vi "烧录座显示界面.vi"(8 "错误输入（无错误）":errorcluster, 10 "界面切换队列":refnum<queue>, 11 "VISA资源名称输入":refnum<visa-resource-name>) -> (0 "错误输出":errorcluster, 3 "VISA资源名称输出":refnum<visa-resource-name>)   [LabVIEW 2018]
panel:
  out "毫秒计时值":u32
  in  "枚举":T1(ring)
  in  "选项卡控件":enum32{"选项卡 1", "选项卡 2"}(tab)
  out "烧录座设定界面":bool
  out "读DDT32250+写R890":dbl
  out "读DDT32252+写R891":dbl
  out "读DDT32254+写R892":dbl
  out "读DDT32256+写R893":dbl
  out "读DDT32258+写R894":dbl
  out "读DDT32260+写R895":dbl
  out "读DDT32262+写R896":dbl
  out "读DDT32264+写R897":dbl
  out "读DDT32266+写R898":dbl
  out "读DDT32268+写R899":dbl
  out "读DDT32270+写R89A":dbl
  out "读DDT32272+写R89B":dbl
  out "读DDT32274+写R89C":dbl
  out "读DDT32276+写R89D":dbl
  out "读DDT32278+写R89E":dbl
  out "读DDT32280+写R89F":dbl
  out "DDT90356":dbl
  out "DDT90348":dbl
  out "自动界面":bool
  out "手动界面":bool
  out "参数界面":bool
  out "IO界面":bool
  out "产品界面":bool
  out "字符串":string
  out "DDT90352":dbl
  out "DDT90360":dbl
  out "通讯周期":dbl
  out "DT1184":T2(ring)
  out "读DDT32200+写R880":dbl
  out "读DDT32202+写R881":dbl
  out "读DDT32204+写R882":dbl
  out "读DDT32206+写R883":dbl
  out "读DDT32208+写R884":dbl
  out "读DDT32210+写R885":dbl
  out "读DDT32212+写R886":dbl
  out "读DDT32214+写R887":dbl
  out "读DDT32216+写R888":dbl
  out "读DDT32218+写R889":dbl
  out "读DDT32220+写R88A":dbl
  out "读DDT32222+写R88B":dbl
  out "读DDT32224+写R88C":dbl
  out "读DDT32226+写R88D":dbl
  out "读DDT32228+写R88E":dbl
  out "读DDT32230+写R88F":dbl
  # "X"
  # "Z1"
  # "Z2"
  # "Y"
  # "1"
  # "2"
  # "3"
  # "4"
  # "5"
  # "6"
  # "7"
  # "8"
  # "9"
  # "10"
  # "12"
  # "14"
  # "15"
  # "16"
  # "11"
  # "13"
  # "烧录座当前OK数量"
  # "鼠标点击数值框清零"
  # "1"
  # "2"
  # "3"
  # "4"
  # "5"
  # "6"
  # "7"
  # "8"
  # "9"
  # "10"
  # "12"
  # "14"
  # "15"
  # "16"
  # "11"
  # "13"
  # "烧录座当前NG数量"
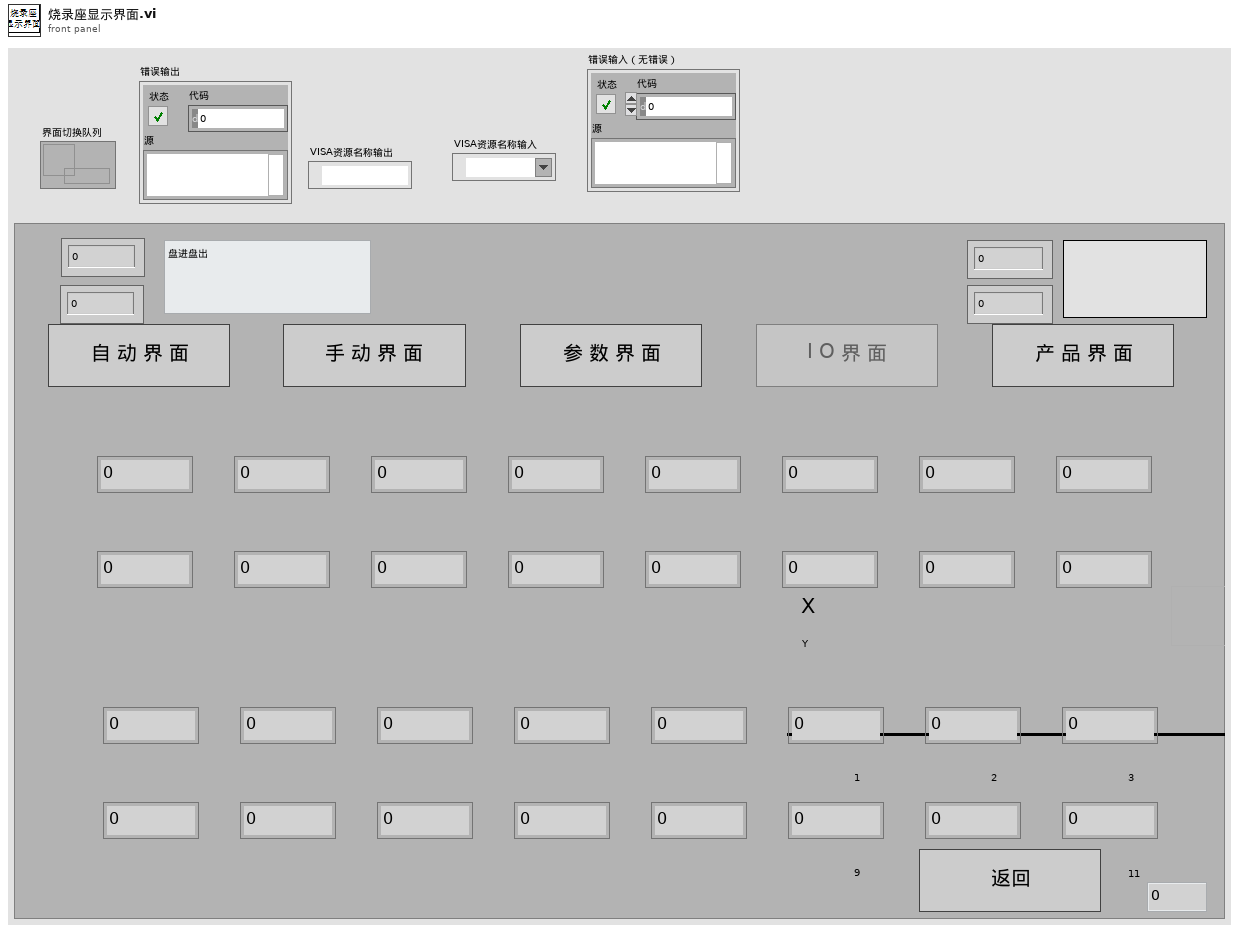
[diagram p1: front panel]
types:
  T1 = enum16{"读初始化", "读DDT32230", "读DDT32220+5", "读DDT32210+5", "读DDT32200+5", "读DDT32280", "读DDT32270+5", "读DDT32260+5", "读DDT32250+5", "读DDT90356", "读DT1184", "读DDT90348", ""}
  T2 = enum16{"盘进盘出", "卷进卷出", "盘进卷出", "管进盘出", "管进卷出", "卷进盘出", ""}
  T3 = enum8{"Enabled", "Disabled", "Disabled and Grayed Out"}
  T4 = typedef "数据簇.ctl" = cluster{"字符串":string, "数值":i32, "布尔":bool}
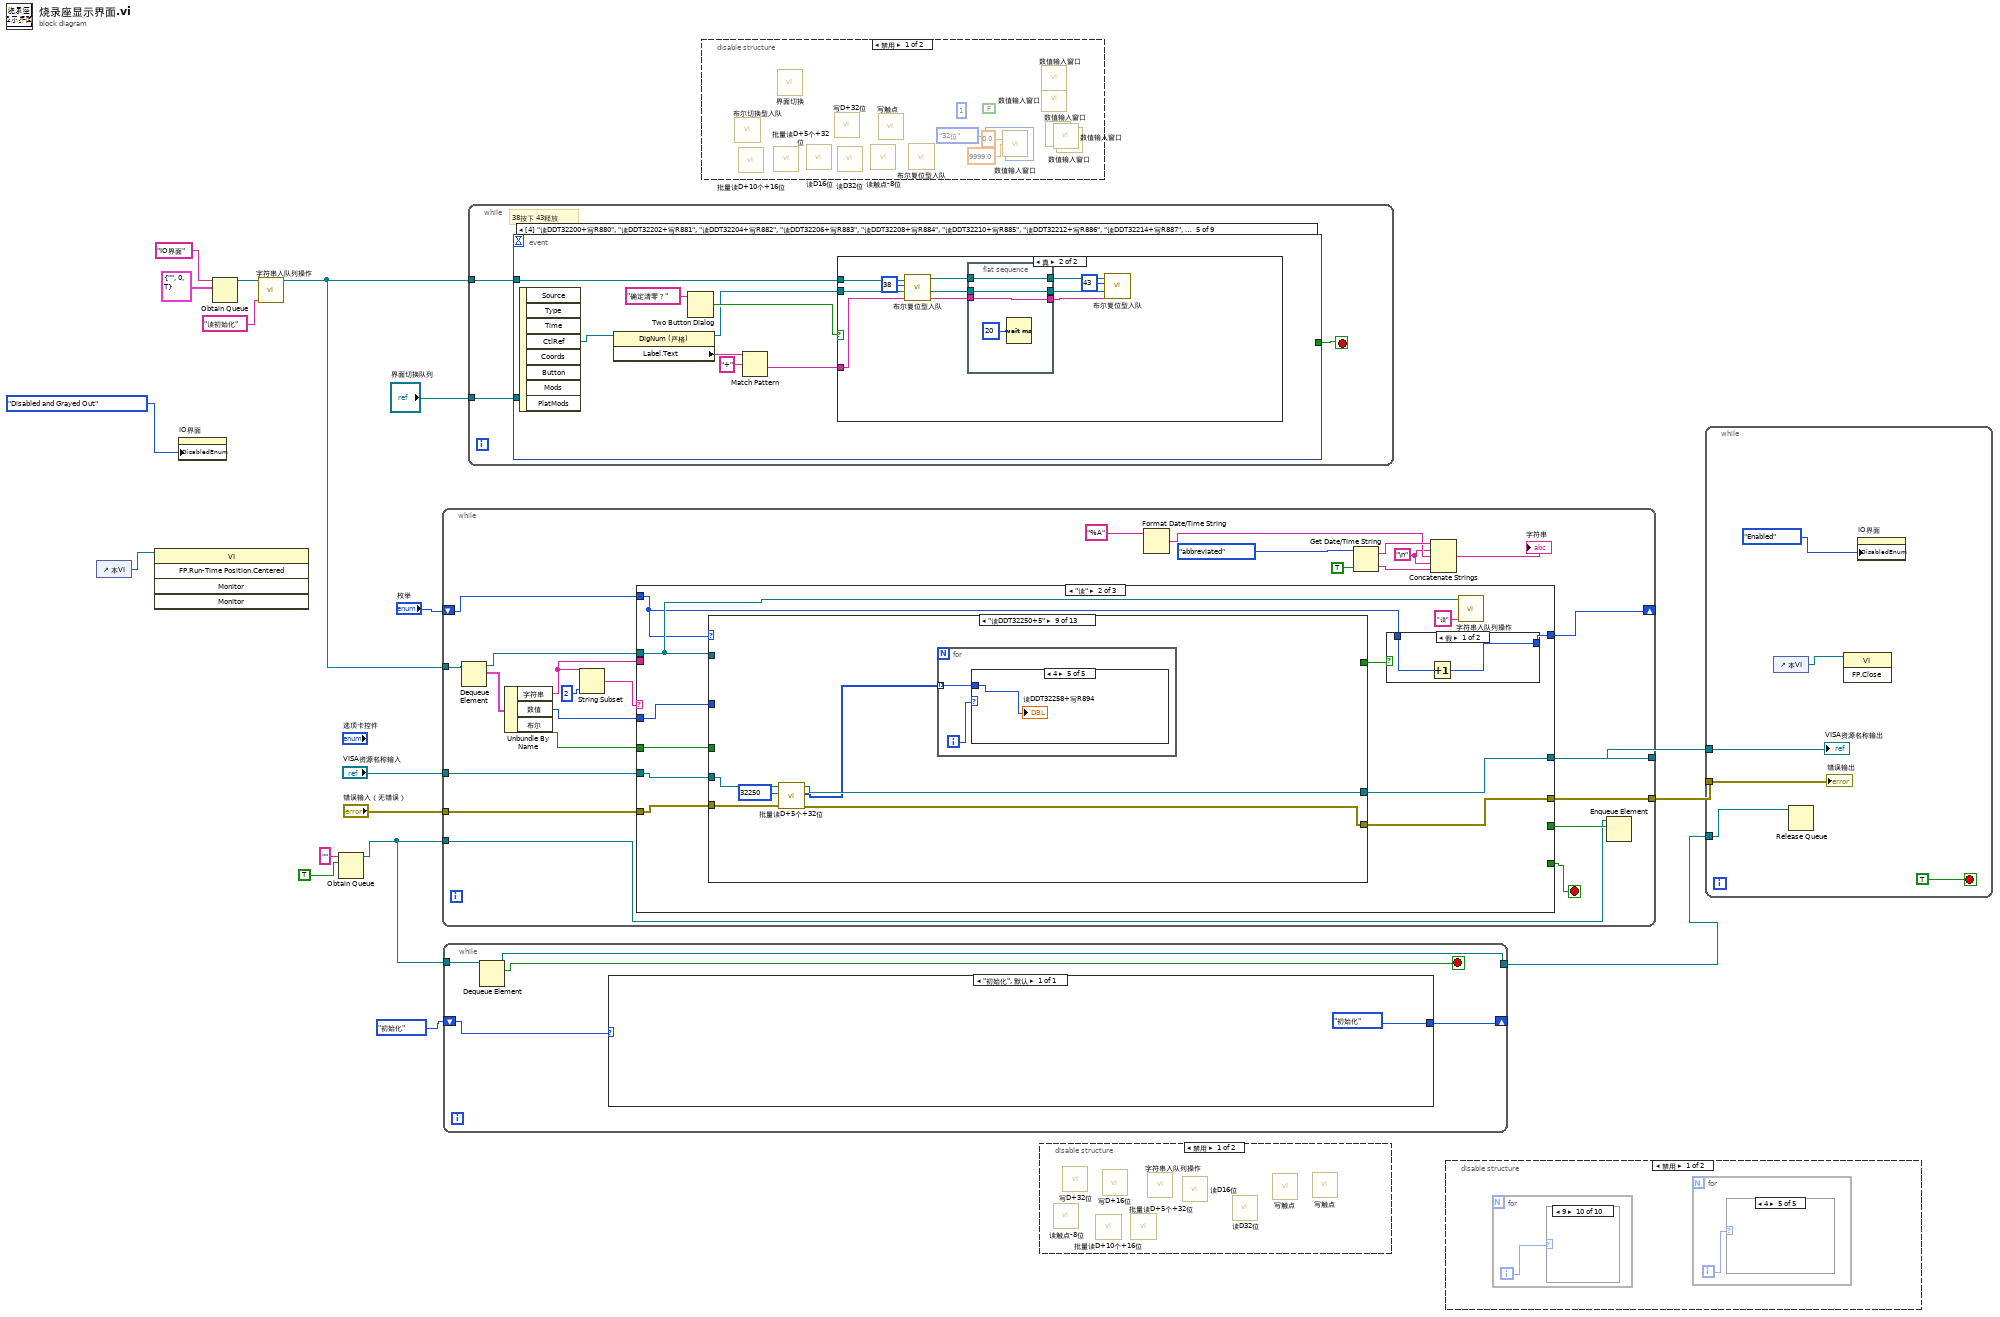
[diagram p0: block diagram]
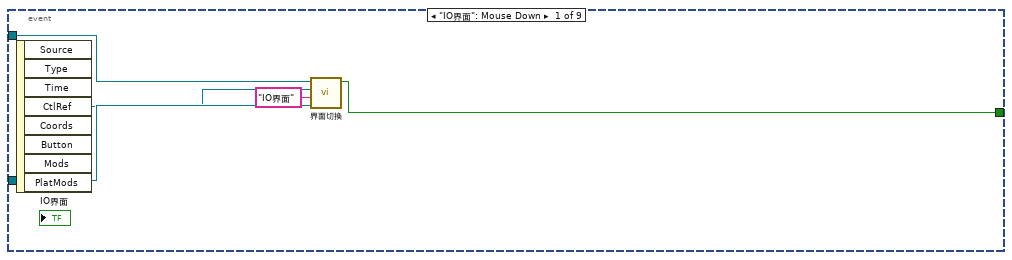
[diagram p18: hidden frame]
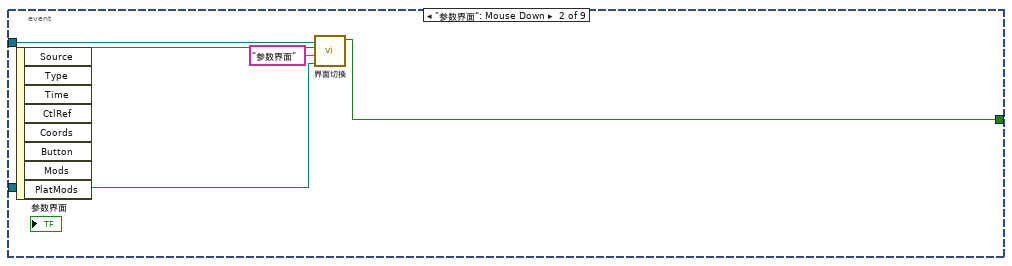
[diagram p19: hidden frame]
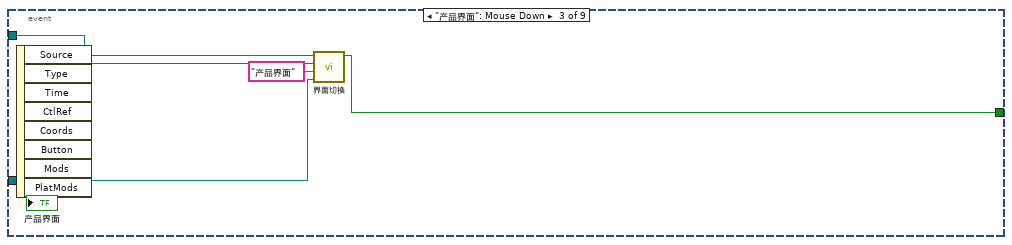
[diagram p20: hidden frame]
diagram:
  n1 = control-ref of="本VI"() -> (w1:refnum<vi>)
  n2 = invoke class="VI" method="FP.Run-Time Position.Centered"(reference=w1) -> ()  [unwired: 4 in, 5 out]
  n3 = property on="IO界面" class="Bool"("DisabledEnum"=T3."Disabled and Grayed Out" ("禁用")) -> ()  [unwired: 2 in, 2 out]
  n4 = Obtain Queue(name (unnamed)="IO界面" ("名称（未命名）"), element data type=T4 {"字符串"="", "数值"=0, "布尔"=TRUE}) -> (queue out=w11:refnum<queue>)  [unwired: 3 in, 2 out]
  n5 = call "字符串入队列操作.vi"("字符消息入队列"="读初始化", "界面切换队列"=w11) -> ("队列输出"=w3:refnum<queue>)  [unwired: 9 in]
  n6 = Obtain Queue(name (unnamed)="" ("名称（未命名）"), element data type=TRUE) -> (queue out=w6:refnum<queue>)  [unwired: 3 in, 2 out]
  n7 = while {
    tunnel: w3 -> [w39]
    tunnel: "VISA资源名称输入" -> [w32]
    tunnel: "错误输入（无错误）" -> [w31]
    tunnel: [w30] -> w13
    tunnel: [w29] -> w12
    shift-right: [w26] -> _
    shift-left: "枚举" -> [w27]
    tunnel: w6 -> [w19]
    stop <- w21 stop-if-true
    w23 = "\n"
    n8 = Dequeue Element(queue=w39) -> (queue out=w36:refnum<queue>, element=w38:T4)  [unwired: 2 in, 2 out]
    n9 = Unbundle By Name(w38) -> ("字符串"=w33:string, "数值"=w35:i32, "布尔"=w34:bool)
    n10 = String Subset(string=w33, length (rest)=2 ("长度（剩余）")) -> (substring=w37:string)  [unwired: 1 in]
    n11 = case shown="\"读\"" w37 {
      selector: w37 -> [w46 _ _]
      tunnel: w36 -> [_ w54 w213]
      tunnel: w35 -> [_ w61 w212]
      tunnel: w34 -> [_ w60 w211]
      tunnel: w33 -> [_ _ w205]
      tunnel: w32 -> [w45 w59 w210]
      tunnel: w31 -> [w44 w58 w209]
      tunnel: [w45 w57 w207] -> w30
      tunnel: [w44 w56 w206] -> w29
      tunnel: [_ _ w208] -> w21
      tunnel: w27 -> [_ w52 _]
      tunnel: [_ w51 _] -> w26
      tunnel: [_ _ w203] -> w20
      frame "", Default {
        n12 = Concatenate Strings("无对应消息分支**" ("消息"), w46, "**" ("字符串"), "读写状态机" ("字符串")) -> (w48:string)
        n13 = One Button Dialog(message=w48) -> ()  [unwired: 1 in, 1 out]
      }
      frame "读" {
        n14 = case shown="\"读DDT32250+5\"" w52 {
          tunnel: w54 -> [_ _ _ _ _ _ _ _ _ _ _ _ _]
          tunnel: w61 -> [_ _ _ _ _ _ _ _ _ _ _ _ _]
          tunnel: w59 -> [w66 w72 w78 w91 w104 w117 w123 w136 w149 w168 w177 w190 w202]
          tunnel: w58 -> [w65 w71 w77 w90 w103 w116 w122 w135 w148 w167 w176 w189 w201]
          tunnel: [w66 w69 w75 w88 w101 w115 w121 w133 w146 w166 w175 w188 w202] -> w57
          tunnel: [w65 w68 w74 w87 w100 w114 w120 w132 w145 w165 w174 w187 w201] -> w56
          tunnel: w60 -> [_ _ _ _ _ _ _ _ _ _ _ _ _]
          tunnel: [_ _ _ _ _ _ _ _ _ _ _ _ TRUE] -> w53
          frame "读初始化" {
            n15 = Tick Count (ms)() -> (millisecond timer value=→"毫秒计时值":u32)
          }
          frame "读DDT32230" {
            n16 = call "读D32位.vi"("error out"=w71, "读取D地址"=32230, "VISA resource name out"=w72) -> ("error IO"=w68:errorcluster, "数值"=→"读DDT32230+写R88F":i32, "VISA resource name out 2"=w69:refnum<visa-resource-name>)  [unwired: 6 in]
          }
          frame "读DDT32220+5" {
            n17 = call "批量读D+5个+32位.vi"("error out"=w77, "读取D地址"=32220, "VISA resource name out"=w78) -> ("error IO"=w74:errorcluster, "数组"=w73:i32[], "VISA resource name out 2"=w75:refnum<visa-resource-name>)  [unwired: 5 in, 1 out]
            n18 = for {
              tunnel: w73 -> [w79] mode=indexing
              i -> [w80]
              n19 = case shown="4" w80 {
                tunnel: w79 -> [w81 w82 w83 w84 w85]
                frame 0, Default {
                  "读DDT32220+写R88A" <- w81
                }
                frame 1 {
                  "读DDT32222+写R88B" <- w82
                }
                frame 2 {
                  "读DDT32224+写R88C" <- w83
                }
                frame 3 {
                  "读DDT32226+写R88D" <- w84
                }
                frame 4 {
                  "读DDT32228+写R88E" <- w85
                }
              }
            }
          }
          frame "读DDT32210+5" {
            n20 = call "批量读D+5个+32位.vi"("error out"=w90, "读取D地址"=32210, "VISA resource name out"=w91) -> ("error IO"=w87:errorcluster, "数组"=w86:i32[], "VISA resource name out 2"=w88:refnum<visa-resource-name>)  [unwired: 5 in, 1 out]
            n21 = for {
              tunnel: w86 -> [w92] mode=indexing
              i -> [w93]
              n22 = case shown="4" w93 {
                tunnel: w92 -> [w94 w95 w96 w97 w98]
                frame 0, Default {
                  "读DDT32210+写R885" <- w94
                }
                frame 1 {
                  "读DDT32212+写R886" <- w95
                }
                frame 2 {
                  "读DDT32214+写R887" <- w96
                }
                frame 3 {
                  "读DDT32216+写R888" <- w97
                }
                frame 4 {
                  "读DDT32218+写R889" <- w98
                }
              }
            }
          }
          frame "读DDT32200+5" {
            n23 = call "批量读D+5个+32位.vi"("error out"=w103, "读取D地址"=32200, "VISA resource name out"=w104) -> ("error IO"=w100:errorcluster, "数组"=w99:i32[], "VISA resource name out 2"=w101:refnum<visa-resource-name>)  [unwired: 5 in, 1 out]
            n24 = for {
              tunnel: w99 -> [w105] mode=indexing
              i -> [w106]
              n25 = case shown="4" w106 {
                tunnel: w105 -> [w107 w108 w109 w110 w111]
                frame 0, Default {
                  "读DDT32200+写R880" <- w107
                }
                frame 1 {
                  "读DDT32202+写R881" <- w108
                }
                frame 2 {
                  "读DDT32204+写R882" <- w109
                }
                frame 3 {
                  "读DDT32206+写R883" <- w110
                }
                frame 4 {
                  "读DDT32208+写R884" <- w111
                }
              }
            }
          }
          frame "读DDT32280" {
            n26 = call "读D32位.vi"("error out"=w116, "读取D地址"=32280, "VISA resource name out"=w117) -> ("error IO"=w114:errorcluster, "数值"=→"读DDT32280+写R89F":i32, "VISA resource name out 2"=w115:refnum<visa-resource-name>)  [unwired: 6 in]
          }
          frame "读DDT32270+5" {
            n27 = call "批量读D+5个+32位.vi"("error out"=w122, "读取D地址"=32270, "VISA resource name out"=w123) -> ("error IO"=w120:errorcluster, "数组"=w118:i32[], "VISA resource name out 2"=w121:refnum<visa-resource-name>)  [unwired: 5 in, 1 out]
            n28 = for {
              tunnel: w118 -> [w124] mode=indexing
              i -> [w125]
              n29 = case shown="4" w125 {
                tunnel: w124 -> [w126 w127 w128 w129 w130]
                frame 0, Default {
                  "读DDT32270+写R89A" <- w126
                }
                frame 1 {
                  "读DDT32272+写R89B" <- w127
                }
                frame 2 {
                  "读DDT32274+写R89C" <- w128
                }
                frame 3 {
                  "读DDT32276+写R89D" <- w129
                }
                frame 4 {
                  "读DDT32278+写R89E" <- w130
                }
              }
            }
          }
          frame "读DDT32260+5" {
            n30 = call "批量读D+5个+32位.vi"("error out"=w135, "读取D地址"=32260, "VISA resource name out"=w136) -> ("error IO"=w132:errorcluster, "数组"=w131:i32[], "VISA resource name out 2"=w133:refnum<visa-resource-name>)  [unwired: 5 in, 1 out]
            n31 = for {
              tunnel: w131 -> [w137] mode=indexing
              i -> [w138]
              n32 = case shown="4" w138 {
                tunnel: w137 -> [w139 w140 w141 w142 w143]
                frame 0, Default {
                  "读DDT32260+写R895" <- w139
                }
                frame 1 {
                  "读DDT32262+写R896" <- w140
                }
                frame 2 {
                  "读DDT32264+写R897" <- w141
                }
                frame 3 {
                  "读DDT32266+写R898" <- w142
                }
                frame 4 {
                  "读DDT32268+写R899" <- w143
                }
              }
            }
          }
          frame "读DDT32250+5" {
            n33 = call "批量读D+5个+32位.vi"("error out"=w148, "读取D地址"=32250, "VISA resource name out"=w149) -> ("error IO"=w145:errorcluster, "数组"=w144:i32[], "VISA resource name out 2"=w146:refnum<visa-resource-name>)  [unwired: 5 in, 1 out]
            n34 = for {
              tunnel: w144 -> [w150] mode=indexing
              i -> [w151]
              n35 = case shown="4" w151 {
                tunnel: w150 -> [w152 w153 w154 w155 w156]
                frame 0, Default {
                  "读DDT32250+写R890" <- w152
                }
                frame 1 {
                  "读DDT32252+写R891" <- w153
                }
                frame 2 {
                  "读DDT32254+写R892" <- w154
                }
                frame 3 {
                  "读DDT32256+写R893" <- w155
                }
                frame 4 {
                  "读DDT32258+写R894" <- w156
                }
              }
            }
          }
          frame "读DDT90356" {
            n36 = call "批量读D+5个+32位.vi"("error out"=w167, "读取D地址"=90356, "VISA resource name out"=w168) -> ("error IO"=w165:errorcluster, "数组"=w171:i32[], "VISA resource name out 2"=w166:refnum<visa-resource-name>)  [unwired: 5 in, 1 out]
            n37 = Index Array(array=w171, index #1=0 ("索引"), index #2=2 ("索引")) -> (element #1=w164:i32, element #2=w163:i32)
            n38 = To Double Precision Float(number=w164) -> (double precision float=w162:dbl)
            n39 = To Double Precision Float(number=w163) -> (double precision float=w159:dbl)
            n40 = Divide(x=w162, y=100.0) -> (x/y=→"DDT90356":dbl)
            n41 = Divide(x=w159, y=100.0) -> (x/y=→"DDT90360":dbl)
          }
          frame "读DT1184" {
            n42 = call "读D16位.vi"("error out"=w176, "读取D地址"=1184, "VISA resource name out"=w177) -> ("error IO"=w174:errorcluster, "数值"=→"DT1184":u32, "VISA resource name out 2"=w175:refnum<visa-resource-name>)  [unwired: 5 in, 1 out]
          }
          frame "读DDT90348" {
            n43 = call "批量读D+5个+32位.vi"("error out"=w189, "读取D地址"=90348, "VISA resource name out"=w190) -> ("error IO"=w187:errorcluster, "数组"=w194:i32[], "VISA resource name out 2"=w188:refnum<visa-resource-name>)  [unwired: 5 in, 1 out]
            n44 = Index Array(array=w194, index #1=0 ("索引"), index #2=2 ("索引")) -> (element #1=w186:i32, element #2=w185:i32)
            n45 = To Double Precision Float(number=w185) -> (double precision float=w180:dbl)
            n46 = To Double Precision Float(number=w186) -> (double precision float=w184:dbl)
            n47 = Divide(x=w180, y=100.0) -> (x/y=→"DDT90352":dbl)
            n48 = Divide(x=w184, y=100.0) -> (x/y=→"DDT90348":dbl)
          }
          frame "" {
            n49 = local read "毫秒计时值"() -> (w198:u32)
            n50 = Tick Count (ms)() -> (millisecond timer value=w199:u32)
            n51 = Subtract(x=w199, y=w198) -> (x-y=w197:u32)
            n52 = Divide(x=w197, y=u32 1000) -> (x/y=→"通讯周期":dbl)
          }
        }
        n53 = case shown="假" w53 {
          tunnel: w52 -> [w63 _]
          tunnel: [w62 _] -> w51
          frame False {
            n54 = Increment(x=w63) -> (x+1=w62:T1)
          }
          frame True {
          }
        }
        n55 = call "字符串入队列操作.vi"("字符消息入队列"="读", "界面切换队列"=w54) -> ()  [unwired: 9 in, 1 out]
      }
      frame "写" {
        n56 = call "状态匹配.vi"("输入状态"=w205) -> ("输出状态"=w204:string)  [unwired: 10 in]
        n57 = case shown="\"写退出\"" w204 {
          selector: w204 -> [w216 _ _ _ _]
          tunnel: w213 -> [_ _ _ _ w256]
          tunnel: w212 -> [_ w222 w239 _ _]
          tunnel: w211 -> [_ _ _ w250 _]
          tunnel: w210 -> [w215 w232 w243 w255 w261]
          tunnel: w209 -> [w214 w231 w242 w254 w260]
          tunnel: [_ _ _ _ w259] -> w208
          tunnel: [w215 w230 w241 w253 w261] -> w207
          tunnel: [w214 w229 w240 w252 w260] -> w206
          tunnel: w205 -> [_ w221 w233 w244 _]
          tunnel: [_ _ _ _ w259] -> w203
          frame "", Default {
            n58 = Concatenate Strings("无对应消息分支**" ("消息"), w216, "**" ("字符串"), "写状态机" ("字符串")) -> (w220:string)
            n59 = One Button Dialog(message=w220) -> ()  [unwired: 1 in, 1 out]
          }
          frame "写DT" {
            n60 = String Length(string=w221) -> (length=w227:i32)
            n61 = Subtract(x=w227, y=4) -> (x-y=w225:i32)
            n62 = String Subset(string=w221, offset (0)=4 ("偏移量(0)"), length (rest)=w225) -> (substring=w224:string)
            n63 = Decimal String To Number(string=w224) -> (number=w223:i32)  [unwired: 2 in, 1 out]
            n64 = call "写D+16位.vi"("error out"=w231, "输入数值"=w222, "输入地址D"=w223, "VISA resource name out"=w232) -> ("error out 2"=w229:errorcluster, "VISA resource name out 2"=w230:refnum<visa-resource-name>)  [unwired: 3 in, 3 out]
          }
          frame "写DDT" {
            n65 = String Length(string=w233) -> (length=w237:i32)
            n66 = Subtract(x=w237, y=5) -> ()  [unwired: 1 out]
            n67 = String Subset(string=w233, offset (0)=5 ("偏移量(0)")) -> (substring=w234:string)  [unwired: 1 in]
            n68 = Decimal String To Number(string=w234) -> (number=w235:i32)  [unwired: 2 in, 1 out]
            n69 = call "写D+32位.vi"("error out"=w242, "输入数值"=w239, "输入地址D"=w235, "VISA resource name out"=w243) -> ("error out 2"=w240:errorcluster, "VISA resource name out 2"=w241:refnum<visa-resource-name>)  [unwired: 4 in, 2 out]
          }
          frame "写R" {
            n70 = String Length(string=w244) -> (length=w248:i32)
            n71 = Subtract(x=w248, y=3) -> (x-y=w246:i32)
            n72 = String Subset(string=w244, offset (0)=3 ("偏移量(0)"), length (rest)=w246) -> (substring=w245:string)
            n73 = call "写触点.vi"("布尔"=w250, "error out"=w254, "触点类型"="R", "写入起始地址"=w245, "VISA resource name out"=w255) -> ("error IO"=w252:errorcluster, "VISA resource name out 2"=w253:refnum<visa-resource-name>)  [unwired: 4 in, 1 out]
          }
          frame "写退出" {
            w259 = TRUE
            n74 = Flush Queue(queue=w256) -> (queue out=w257:refnum<queue>, error out=w258:errorcluster)  [unwired: 1 in, 1 out]
            n75 = Release Queue(queue=w257, error in (no error)=w258) -> ()  [unwired: 1 in, 3 out]
          }
        }
      }
    }
    n76 = Format Date/Time String(time format string (%c)="%A" ("时间格式字符串(%c)")) -> (date/time string=w24:string)  [unwired: 2 in]
    n77 = Get Date/Time String(date format (0)=enum16{"short", "long", "abbreviated"}."abbreviated" ("日期格式(0)"), want seconds? (F)=TRUE ("需要秒？(F)")) -> (date string=w41:string, time string=w22:string)  [unwired: 1 in]
    n78 = Concatenate Strings(w41, w23, w24, w23, w22) -> (→"字符串":string)
    n79 = Enqueue Element(queue=w19, element=w20) -> ()  [unwired: 2 in, 3 out]
  }
  n80 = while {
    shift-right: [w265] -> _
    shift-left: enum16{"初始化"}."初始化" -> [w266]
    tunnel: w6 -> [w264]
    tunnel: [w262] -> w5
    stop <- w263 stop-if-true
    n81 = Dequeue Element(queue=w264) -> (queue out=w262:refnum<queue>, element=w263:bool)  [unwired: 2 in, 2 out]
    n82 = case shown="\"初始化\", 默认" w266 {
      tunnel: [enum16{"初始化"}."初始化"] -> w265
      frame "初始化", Default {
      }
    }
  }
  n83 = while {
    tunnel: w3 -> [w269]
    tunnel: "界面切换队列" -> [w268]
    stop <- w270 stop-if-true
    # "38按下 43释放"
    n84 = event shown="[4] \"读DDT32200+写R880\", \"读DDT32202+写R881\", \"读DDT32204+写R882\", \"读DDT32206+写R883\", \"读DDT32208+写R884\", \"读DDT32210+写R885\", \"读DDT32212+写R886\", \"读DDT32214+写R887\", \"读DDT32216+写R888\", \"读DDT32218+写R889\", \"读DDT32220+写R88A\", \"读DDT32222+写R88B\", \"读DDT32224+写R88C\", \"读DDT32226+写R88D\", \"读DDT32228+写R88E\", \"读DDT32230+写R88F\", \"读DDT32280+写R89F\", \"读DDT32278+写R89E\", \"读DDT32276+写R89D\", \"读DDT32274+写R89C\", \"读DDT32272+写R89B\", \"读DDT32270+写R89A\", \"读DDT32268+写R899\", \"读DDT32266+写R898\", \"读DDT32264+写R897\", \"读DDT32262+写R896\", \"读DDT32260+写R895\", \"读DDT32258+写R894\", \"读DDT32256+写R893\", \"读DDT32254+写R892\", \"读DDT32252+写R891\", \"读DDT32250+写R890\": 鼠标按下" {
      selector: _ -> [_ _ _ _ _ _ _ _ _]
      dyn-events: _ -> [_ _ _ _ _ _ _ _ _]
      timeout: _ -> [_ _ _ _ _ _ _ _ _]
      tunnel: [w274 w276 w281 w289 _ w314 w319 _ w326] -> w270
      tunnel: w269 -> [w275 w280 w285 w290 w293 w318 w323 _ w325]
      tunnel: w268 -> [w273 w279 w284 w288 _ w317 w322 _ w324]
      event "IO界面": Mouse Down {
        n85 = event-data() -> ("CtlRef"=w272:refnum<vi>)  [unwired: 1 in, 7 out]
        n86 = call "界面切换.vi"("界面切换队列输入"=w273, "切换界面名称输入"="IO界面", "Bool引用句柄"=w272, "状态转移输入"=w275) -> ("布尔"=w274:bool)  [unwired: 7 in]
      }
      event "参数界面": Mouse Down {
        n87 = event-data() -> ("CtlRef"=w278:refnum<vi>)  [unwired: 1 in, 7 out]
        n88 = call "界面切换.vi"("界面切换队列输入"=w279, "切换界面名称输入"="参数界面", "Bool引用句柄"=w278, "状态转移输入"=w280) -> ("布尔"=w276:bool)  [unwired: 7 in]
      }
      event "产品界面": Mouse Down {
        n89 = event-data() -> ("CtlRef"=w283:refnum<vi>)  [unwired: 1 in, 7 out]
        n90 = call "界面切换.vi"("界面切换队列输入"=w284, "切换界面名称输入"="产品界面", "Bool引用句柄"=w283, "状态转移输入"=w285) -> ("布尔"=w281:bool)  [unwired: 7 in]
      }
      event "烧录座设定界面": Mouse Down {
        n91 = event-data() -> ("CtlRef"=w287:refnum<vi>)  [unwired: 1 in, 7 out]
        n92 = call "界面切换.vi"("界面切换队列输入"=w288, "切换界面名称输入"="烧录座设定界面", "Bool引用句柄"=w287, "状态转移输入"=w290) -> ("布尔"=w289:bool)  [unwired: 7 in]
      }
      event "读DDT32200+写R880", "读DDT32202+写R881", "读DDT32204+写R882", "读DDT32206+写R883", "读DDT32208+写R884", "读DDT32210+写R885", "读DDT32212+写R886", "读DDT32214+写R887", "读DDT32216+写R888", "读DDT32218+写R889", "读DDT32220+写R88A", "读DDT32222+写R88B", "读DDT32224+写R88C", "读DDT32226+写R88D", "读DDT32228+写R88E", "读DDT32230+写R88F", "读DDT32280+写R89F", "读DDT32278+写R89E", "读DDT32276+写R89D", "读DDT32274+写R89C", "读DDT32272+写R89B", "读DDT32270+写R89A", "读DDT32268+写R899", "读DDT32266+写R898", "读DDT32264+写R897", "读DDT32262+写R896", "读DDT32260+写R895", "读DDT32258+写R894", "读DDT32256+写R893", "读DDT32254+写R892", "读DDT32252+写R891", "读DDT32250+写R890": Mouse Down {
        n93 = event-data() -> ("CtlRef"=w296:refnum<vi>)  [unwired: 1 in, 7 out]
        n94 = property class="DigNum (严格)"(reference=w296) -> (reference out=w292:refnum<vi>, "Label.Text"=w295:string)  [unwired: 1 in, 1 out]
        n95 = Two Button Dialog(message="确定清零？" ("消息")) -> (T button?=w297:bool)  [unwired: 2 in]
        n96 = Match Pattern(string=w295, regular expression="+" ("正则表达式")) -> (after substring=w291:string)  [unwired: 1 in, 3 out]
        n97 = case shown="真" w297 {
          tunnel: w293 -> [_ w309]
          tunnel: w292 -> [_ w308]
          tunnel: w291 -> [_ w306]
          frame False {
          }
          frame True {
            n98 = call "布尔复位型入队.vi"("队列输入"=w309, "数值"=38, "控件引用"=w308, "字符消息入队列"=w306) -> ("队列输出"=w305:refnum<queue>, "控件引用 2"=w304:refnum<vi>, "字符消息出队列"=w303:string)  [unwired: 2 in]
            n99 = flat-sequence {
              tunnel: w305 -> [w313]
              tunnel: w304 -> [w312]
              tunnel: w303 -> [w311]
              tunnel: [w313] -> w302
              tunnel: [w312] -> w301
              tunnel: [w311] -> w300
              frame #0 {
                n100 = Wait (ms)(milliseconds to wait=u32 20 ("等待时间（毫秒）")) -> ()  [unwired: 1 out]
              }
            }
            n101 = call "布尔复位型入队.vi"("队列输入"=w302, "数值"=43, "控件引用"=w301, "字符消息入队列"=w300) -> ()  [unwired: 2 in, 3 out]
          }
        }
      }
      event "手动界面": Mouse Down {
        n102 = event-data() -> ("CtlRef"=w316:refnum<vi>)  [unwired: 1 in, 7 out]
        n103 = call "界面切换.vi"("界面切换队列输入"=w317, "切换界面名称输入"="手动界面", "Bool引用句柄"=w316, "状态转移输入"=w318) -> ("布尔"=w314:bool)  [unwired: 7 in]
      }
      event "自动界面": Mouse Down {
        n104 = event-data() -> ("CtlRef"=w321:refnum<vi>)  [unwired: 1 in, 7 out]
        n105 = call "界面切换.vi"("界面切换队列输入"=w322, "切换界面名称输入"="自动界面", "Bool引用句柄"=w321, "状态转移输入"=w323) -> ("布尔"=w319:bool)  [unwired: 7 in]
      }
      event Timeout {
        n106 = event-data() -> ()  [unwired: 1 in, 3 out]
      }
      event Panel Close? {
        n107 = event-data() -> ()  [unwired: 1 in, 4 out]
        n108 = Two Button Dialog(message="确定退出程序？" ("消息")) -> (T button?=w327:bool)  [unwired: 2 in]
        n109 = case shown="真" w327 {
          tunnel: [_ TRUE] -> w326
          tunnel: w325 -> [_ w332]
          tunnel: w324 -> [_ w331]
          frame False {
          }
          frame True {
            n110 = call "字符串入队列操作.vi"("字符消息入队列"="退出", "界面切换队列"=w331) -> ()  [unwired: 9 in, 1 out]
            n111 = call "字符串入队列操作.vi"("字符消息入队列"="写退出", "界面切换队列"=w332) -> ()  [unwired: 9 in, 1 out]
          }
        }
        n112 = event-data("Discard?"=TRUE ("放弃？")) -> ()  [unwired: 1 in, 1 out]
      }
    }
  }
  n113 = disable-structure shown="禁用" {
    frame Disabled {
      (unwired) u32 1 ("转换比例")
      (unwired) FALSE ("忽略数值上下限")
      n114 = call "布尔切换型入队.vi"() -> ()  [unwired: 12 in]
      n115 = call "批量读D+10个+16位.vi"() -> ()  [unwired: 8 in, 4 out]
      n116 = call "批量读D+5个+32位.vi"() -> ()  [unwired: 8 in, 4 out]
      n117 = call "界面切换.vi"() -> ()  [unwired: 11 in, 1 out]
      n118 = call "读D16位.vi"() -> ()  [unwired: 8 in, 4 out]
      n119 = call "写D+32位.vi"() -> ()  [unwired: 8 in, 4 out]
      n120 = call "读D32位.vi"() -> ()  [unwired: 9 in, 3 out]
      n121 = call "读触点-8位.vi"() -> ()  [unwired: 8 in, 4 out]
      n122 = call "写触点.vi"() -> ()  [unwired: 9 in, 3 out]
      n123 = call "布尔复位型入队.vi"() -> ()  [unwired: 6 in, 3 out]
      n124 = call "数值输入窗口.vi"("输入下限"=0.0, "输入上限"=9999.0, "数据类型"=enum16{"32位", "16位"}."32位") -> ("转换比例"=w338:u32)  [unwired: 9 in, 3 out]
      n125 = call "数值输入窗口.vi"() -> ()  [unwired: 13 in, 3 out]
      n126 = call "数值输入窗口.vi"() -> ()  [unwired: 13 in, 3 out]
      n127 = call "数值输入窗口.vi"() -> ()  [unwired: 13 in, 3 out]
      n128 = call "数值输入窗口.vi"() -> ()  [unwired: 13 in, 3 out]
      n129 = call "数值输入窗口.vi"() -> ()  [unwired: 13 in, 3 out]
    }
    frame Enabled {
    }
  }
  n130 = disable-structure shown="禁用" {
    frame Disabled {
      n131 = call "读触点-8位.vi"() -> ()  [unwired: 8 in, 4 out]
      n132 = call "写D+32位.vi"() -> ()  [unwired: 8 in, 4 out]
      n133 = call "批量读D+10个+16位.vi"() -> ()  [unwired: 8 in, 4 out]
      n134 = call "写D+16位.vi"() -> ()  [unwired: 7 in, 5 out]
      n135 = call "批量读D+5个+32位.vi"() -> ()  [unwired: 8 in, 4 out]
      n136 = call "字符串入队列操作.vi"() -> ()  [unwired: 11 in, 1 out]
      n137 = call "读D16位.vi"() -> ()  [unwired: 8 in, 4 out]
      n138 = call "读D32位.vi"() -> ()  [unwired: 9 in, 3 out]
      n139 = call "写触点.vi"() -> ()  [unwired: 9 in, 3 out]
      n140 = call "写触点.vi"() -> ()  [unwired: 9 in, 3 out]
    }
    frame Enabled {
    }
  }
  n141 = disable-structure shown="禁用" {
    frame Disabled {
      n142 = for {
        i -> [w340]
        n143 = case shown="9" w340 {
          frame 0, Default {
          }
          frame 1 {
          }
          frame 2 {
          }
          frame 3 {
          }
          frame 4 {
          }
          frame 5 {
          }
          frame 6 {
          }
          frame 7 {
          }
          frame 8 {
          }
          frame 9 {
          }
        }
      }
      n144 = for {
        i -> [w339]
        n145 = case shown="4" w339 {
          frame 0, Default {
          }
          frame 1 {
          }
          frame 2 {
          }
          frame 3 {
          }
          frame 4 {
          }
        }
      }
    }
    frame Enabled {
    }
  }
  n146 = while {
    tunnel: w13 -> [w344]
    tunnel: w12 -> [w343]
    tunnel: w5 -> [w342]
    stop <- TRUE stop-if-true
    n147 = control-ref of="本VI"() -> (w345:refnum<vi>)
    n148 = Release Queue(queue=w342) -> ()  [unwired: 2 in, 3 out]
    n149 = invoke class="VI" method="FP.Close"(reference=w345) -> ()  [unwired: 2 in, 3 out]
    n150 = property on="IO界面" class="Bool"("DisabledEnum"=T3."Enabled" ("禁用")) -> ()  [unwired: 2 in, 2 out]
    "VISA资源名称输出" <- w344
    "错误输出" <- w343
  }
